vi "Add Separator.vi"(8 "error in (no error)":errorcluster, 10 "Icon Index (Next)":i32=-1, 11 "Toolbar Control in":refnum<class "Toolbar Control.lvclass">) -> (0 "error out":errorcluster, 3 "Toolbar Control out":refnum<class "Toolbar Control.lvclass">)   [LabVIEW 2011, in "Toolbar Control.lvclass"]
doc: "This VI will add the image of a separator to the <B>Toolbar Control in</B> at the available location or if specified by <B>Icon Index (Next)</B>.\n\n-------------\nDeveloped by Brian Hoover (hooovahh)"
uses:
  Toolbar Control.lvclass
  Toolbar Control.lvclass/Toolbar Control.ctl
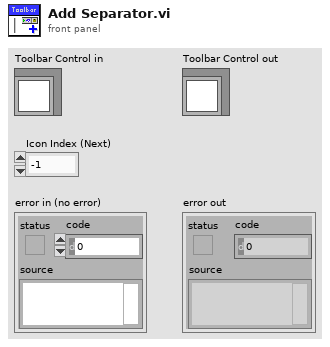
[diagram p1: front panel]
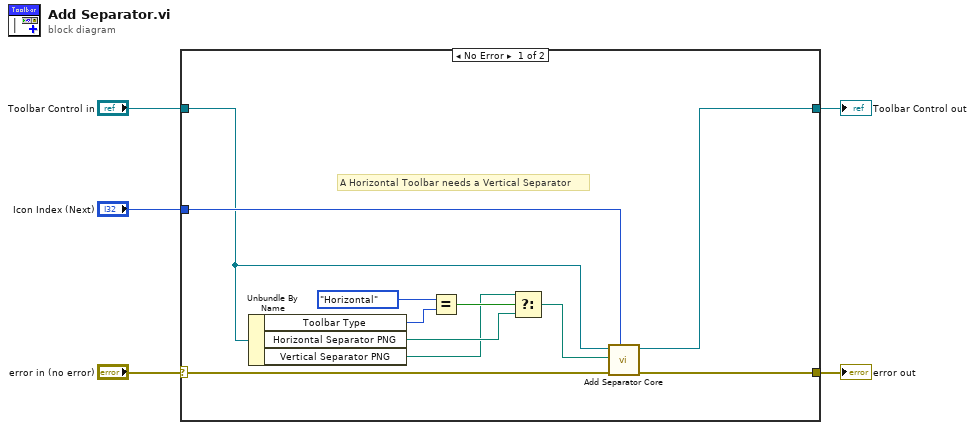
[diagram p0: block diagram]
diagram:
  n1 = case shown="No Error" "error in (no error)" {
    selector: "error in (no error)" -> [w15 w18]
    tunnel: [w14 w18] -> w4
    tunnel: [w12 w17] -> w2
    tunnel: "Toolbar Control in" -> [w13 w17]
    tunnel: "Icon Index (Next)" -> [w16 _]
    frame No Error {
      # "A Horizontal Toolbar needs a Vertical Separator"
      n2 = Unbundle By Name(w13) -> ("Toolbar Type"=w11:enum16{"Horizontal", "Vertical"}, "Horizontal Separator PNG"=w8:path, "Vertical Separator PNG"=w7:path)
      n3 = Equal?(x=enum16{"Horizontal", "Vertical"}."Horizontal", y=w11) -> (x = y?=w9:bool)
      n4 = Select(t=w7, s=w9, f=w8) -> (s? t:f=w6:path)
      n5 = call "Add Separator Core.vi"("Icon Index (Next)"=w16, "error in (no error)"=w15, "Image Path"=w6, "Toolbar Control in"=w13) -> ("error out"=w14:errorcluster, "Toolbar Control out"=w12:refnum<class "Toolbar Control.lvclass">)  [unwired: 6 in]
    }
    frame Error {
    }
  }
  "error out" <- w4
  "Toolbar Control out" <- w2
